vi "SplitOverlay.vi"(8 "dB Max":dbl, 9 "Raw data":cdb[][](array[numeric]), 10 "Doppler Data":dbl[][](graph), 11 "Z Scale":dbl(slide) scale=0.0..80.0) -> (2 "Overlay":i16[][](graph))   [LabVIEW 2022 SP3]
uses:
  <vilib>/Analysis/NI_AALPro.lvlib
panel:
  out "appended array":u32[](array[numeric])
  out "Raw data 3":dbl[][](graph)
  out "Raw data 2":i16[][](graph)
  in  "Grey Scale":u32[](array[colorbox])=[0, 65793, 65793, 131586, 197379, 263172, 328965, 394758, 460551, 526344, 592137, 657930, 723723, 789516, 855309, 921102, 986895, 1052688, 1118481, 1184274, 1250067, 1315860, 1381653, 1447446, 1513239, 1579032, 1644825, 1710618, 1776411, 1842204, 1907997, 1973790, 2039583, 2105376, 2171169, 2236962, 2302755, 2368548, 2434341, 2500134, 2565927, 2631720, 2697513, 2763306, 2829099, 2894892, 2960685, 3026478, 3092271, 3158064, 3223857, 3289650, 3355443, 3421236, 3487029, 3552822, 3618615, 3684408, 3750201, 3815994, 3881787, 3947580, 4013373, 4079166, 4144959, 4210752, 4276545, 4342338, 4408131, 4473924, 4539717, 4605510, 4671303, 4737096, 4802889, 4868682, 4934475, 5000268, 5066061, 5131854, 5197647, 5263440, 5329233, 5395026, 5460819, 5526612, 5592405, 5658198, 5723991, 5789784, 5855577, 5921370, 5987163, 6052956, 6118749, 6184542, 6250335, 6316128, 6381921, 6447714, 6513507, 6579300, 6645093, 6710886, 6776679, 6842472, 6908265, 6974058, 7039851, 7105644, 7171437, 7237230, 7303023, 7368816, 7434609, 7500402, 7566195, 7631988, 7697781, 7763574, 7829367, 7895160, 7960953, 8026746, 8092539, 8158332, 8224125, 8289918, 8355711, 8421504, 8487297, 8553090, 8618883, 8684676, 8750469, 8816262, 8882055, 8947848, 9013641, 9079434, 9145227, 9211020, 9276813, 9342606, 9408399, 9474192, 9539985, 9605778, 9671571, 9737364, 9803157, 9868950, 9934743, 10000536, 10066329, 10132122, 10197915, 10263708, 10329501, 10395294, 10461087, 10526880, 10592673, 10658466, 10724259, 10790052, 10855845, 10921638, 10987431, 11053224, 11119017, 11184810, 11250603, 11316396, 11382189, 11447982, 11513775, 11579568, 11645361, 11711154, 11776947, 11842740, 11908533, 11974326, 12040119, 12105912, 12171705, 12237498, 12303291, 12369084, 12434877, 12500670, 12566463, 12632256, 12698049, 12763842, 12829635, 12895428, 12961221, 13027014, 13092807, 13158600, 13224393, 13290186, 13355979, 13421772, 13487565, 13553358, 13619151, 13684944, 13750737, 13816530, 13882323, 13948116, 14013909, 14079702, 14145495, 14211288, 14277081, 14342874, 14408667, 14474460, 14540253, 14606046, 14671839, 14737632, 14803425, 14869218, 14935011, 15000804, 15066597, 15132390, 15198183, 15263976, 15329769, 15395562, 15461355, 15527148, 15592941, 15658734, 15724527, 15790320, 15856113, 15921906, 15987699, 16053492, 16119285, 16185078, 16250871, 16316664, 16382457, 16448250, 16514043, 16579836, 16645629, 16711680]
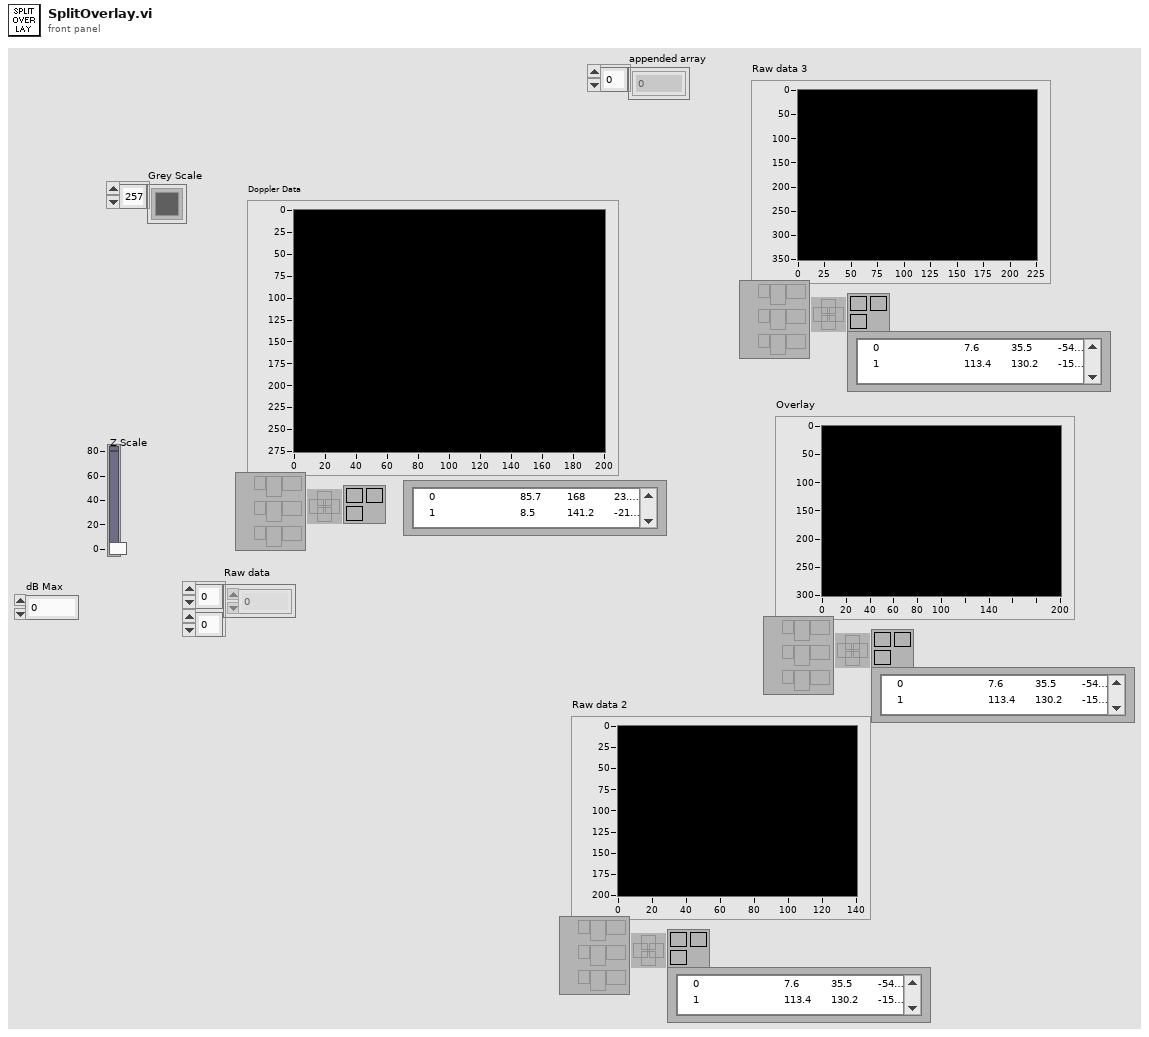
[diagram p1: front panel]
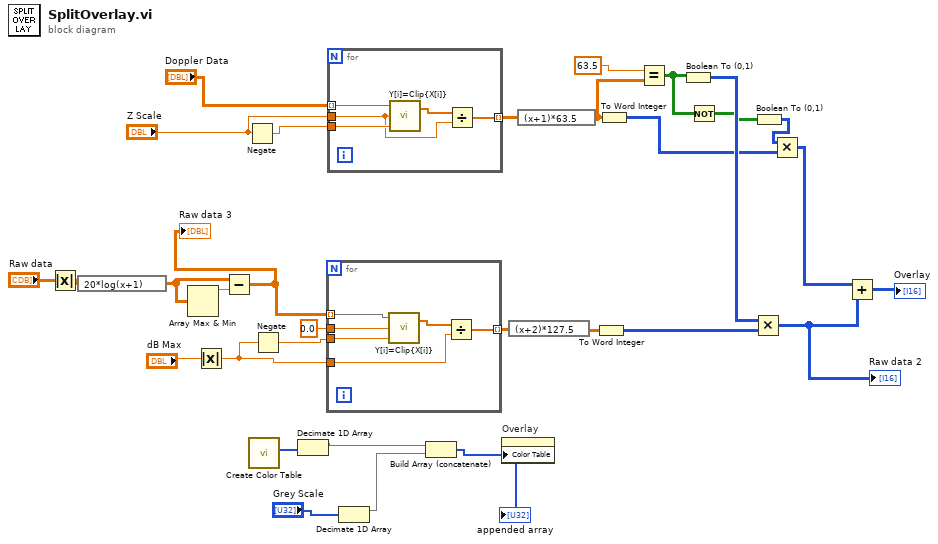
[diagram p0: block diagram]
diagram:
  n1 = Absolute Value(x="Raw data") -> (abs(x)=w7:dbl[][])
  n2 = expression code="20*log(x+1)"(w7) -> (w6:dbl[][])
  n3 = Array Max & Min(array=w6) -> (max value=w19:dbl)  [unwired: 3 out]
  n4 = Absolute Value(x="dB Max") -> (abs(x)=w20:dbl)
  n5 = Subtract(x=w6, y=w19) -> (x-y=w15:dbl[][])
  "Raw data 3" <- w15
  n6 = Negate(x="Z Scale") -> (-x=w31:dbl)
  n7 = call "Create Color Table.vi"() -> ("Color Table"=w4:u32[])  [unwired: 10 in, 1 out]
  n8 = Negate(x=w20) -> (-x=w26:dbl)
  n9 = Decimate 1D Array(w4) -> (w3:u32[])  [unwired: 1 out]
  n10 = for {
    tunnel: w26 -> [w37]
    tunnel: 0.0 ("Z Scale") -> [w35]
    tunnel: [w34] -> w24 mode=indexing
    tunnel: w15 -> [w33] mode=indexing
    tunnel: w20 -> [w32]
    n11 = call <vilib>:"Y[i]=Clip{X[i]}.vi"("lower limit"=w37, "upper limit"=w35, "Input Array"=w33) -> ("Clipped Array"=w36:dbl[])  [unwired: 1 out]
    n12 = Divide(x=w36, y=w32) -> (x/y=w34:dbl[])
  }
  n13 = for {
    tunnel: "Doppler Data" -> [w42] mode=indexing
    tunnel: w31 -> [w41]
    tunnel: "Z Scale" -> [w39]
    tunnel: [w38] -> w23 mode=indexing
    n14 = call <vilib>:"Y[i]=Clip{X[i]}.vi"("lower limit"=w41, "upper limit"=w39, "Input Array"=w42) -> ("Clipped Array"=w40:dbl[])  [unwired: 1 out]
    n15 = Divide(x=w40, y=w39) -> (x/y=w38:dbl[])
  }
  n16 = Decimate 1D Array("Grey Scale") -> (w1:u32[])  [unwired: 1 out]
  n17 = Build Array (concatenate)(w3, w1) -> (w2:u32[])
  "appended array" <- w2
  n18 = property on="Overlay" class="IntGraph (strict)"("Color Table"=w2) -> ()  [unwired: 2 in, 2 out]
  n19 = expression code="(x+2)*127.5"(w24) -> (w25:dbl[][])
  n20 = expression code="(x+1)*63.5"(w23) -> (w14:dbl[][])
  n21 = To Word Integer(number=w25) -> (16bit integer=w17:i16[][])
  n22 = To Word Integer(number=w14) -> (16bit integer=w12:i16[][])
  n23 = Equal?(x=63.5 ("Z Scale"), y=w14) -> (x = y?=w10:bool[][])
  n24 = Boolean To (0,1)(Boolean=w10) -> (0, 1=w13:i16[][])
  n25 = Not(x=w10) -> (.not. x?=w9:bool[][])
  n26 = Multiply(x=w13, y=w17) -> (x*y=w16:i16[][])
  "Raw data 2" <- w16
  n27 = Boolean To (0,1)(Boolean=w9) -> (0, 1=w8:i16[][])
  n28 = Multiply(x=w8, y=w12) -> (x*y=w11:i16[][])
  n29 = Add(x=w11, y=w16) -> (x+y=→"Overlay":i16[][])
